vi "Laser on(SubVI).vi"() -> (0 "error out":errorcluster, 2 "Laser On":bool, 3 "ASG Connection On?":bool)   [LabVIEW 2020]
uses:
  Labview Library/Libraries/ASG8100CY/ASG8X00_x64.dll
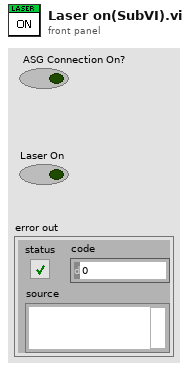
[diagram p1: front panel]
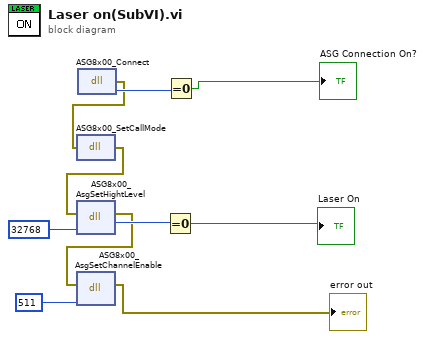
[diagram p0: block diagram]
diagram:
  n1 = dll-call lib="F:/Labview Library/Libraries/ASG8100CY/ASG8X00_x64.dll" fn="ASG8x00_Connect"() -> (error out=w1:errorcluster, "返回类型"=w5:i32)  [unwired: 3 in, 1 out]
  n2 = dll-call lib="F:/Labview Library/Libraries/ASG8100CY/ASG8X00_x64.dll" fn="ASG8x00_SetCallMode"(error in=w1) -> (error out=w2:errorcluster)  [unwired: 3 in, 1 out]
  n3 = dll-call lib="F:/Labview Library/Libraries/ASG8100CY/ASG8X00_x64.dll" fn="ASG8x00_AsgSetHightLevel"(error in=w2, "参数1"=32768) -> (error out=w3:errorcluster, "返回类型"=w9:i32)  [unwired: 3 in, 1 out]
  n4 = dll-call lib="F:/Labview Library/Libraries/ASG8100CY/ASG8X00_x64.dll" fn="ASG8x00_AsgSetChannelEnable"(error in=w3, "参数1"=511) -> (error out=→"error out":errorcluster)  [unwired: 4 in, 1 out]
  n5 = Equal To 0?(x=w9) -> (x = 0?=→"Laser On":bool)
  n6 = Equal To 0?(x=w5) -> (x = 0?=→"ASG Connection On?":bool)
